vi "Read HWND.vi"(8 "error in (no error)":errorcluster, 11 "Container base in":refnum<class "Container base.lvclass">) -> (0 "error out":errorcluster, 2 "HWND":i32, 3 "Container base out":refnum<class "Container base.lvclass">)   [LabVIEW 2016, in "Container base.lvclass"]
uses:
  Container base.lvclass
  Container base.lvclass/Container base.ctl
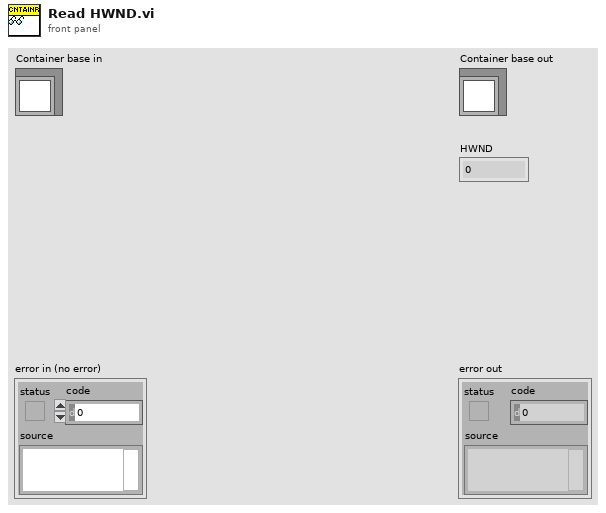
[diagram p1: front panel]
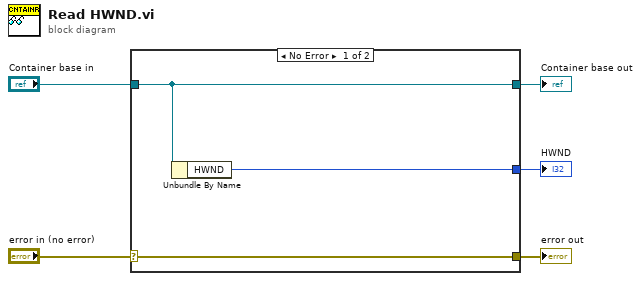
[diagram p0: block diagram]
diagram:
  n1 = case shown="No Error" "error in (no error)" {
    selector: "error in (no error)" -> [w8 w9]
    tunnel: [w8 w9] -> w4
    tunnel: [w7 w10] -> w2
    tunnel: "Container base in" -> [w7 w10]
    tunnel: [w6 _] -> w1
    frame No Error {
      n2 = Unbundle By Name(w7) -> ("HWND"=w6:i32)
    }
    frame Error {
    }
  }
  "error out" <- w4
  "Container base out" <- w2
  "HWND" <- w1
